vi "Practica 10 ITIW31 Tejada.vi"() -> ()   [LabVIEW 2018]
panel:
  out "VAs Requeridos":dbl
  out "VAs Individual":dbl
  in  "WATTS (W)":dbl
  out "Total de VAs\nRequeridos":dbl
  out "Factor de \nCrecimiento\npor años (%)":dbl
  in  "Subtotal":dbl
  out "Total de KVAs\nRequeridos":dbl
  out "VA Requeridos \npor todas las\nEquipos":dbl
  out "VA Individuales\nde las \nEquipos":dbl
  in  "Corriente de las \nEquipos\nen Amperes":dbl
  in  "No. Equipos":dbl
  in  "Voltaje en AC":dbl
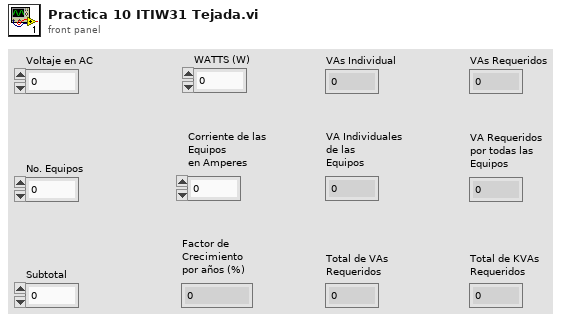
[diagram p1: front panel]
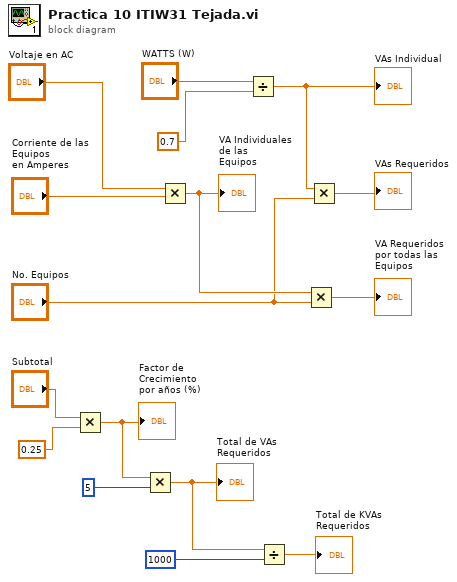
[diagram p0: block diagram]
diagram:
  n1 = Multiply(x="Subtotal", y=0.25) -> (x*y=w7:dbl)
  "Factor de \nCrecimiento\npor años (%)" <- w7
  n2 = Multiply(x=w7, y=5) -> (x*y=w6:dbl)
  "Total de VAs\nRequeridos" <- w6
  n3 = Multiply(x="Voltaje en AC", y="Corriente de las \nEquipos\nen Amperes") -> (x*y=w14:dbl)
  "VA Individuales\nde las \nEquipos" <- w14
  n4 = Divide(x="WATTS (W)", y=0.7) -> (x/y=w3:dbl)
  "VAs Individual" <- w3
  n5 = Divide(x=w6, y=1000) -> (x/y=→"Total de KVAs\nRequeridos":dbl)
  n6 = Multiply(x=w14, y="No. Equipos") -> (x*y=→"VA Requeridos \npor todas las\nEquipos":dbl)
  n7 = Multiply(x=w3, y="No. Equipos") -> (x*y=→"VAs Requeridos":dbl)
